vi "New from bytes.vi"(8 "error in":errorcluster, 11 "bytes":u8[](array[numeric]) format="%x") -> (0 "error out":errorcluster, 2 "output cluster":refnum<class "MsgPackString.lvclass">, 3 "remaining bytes":u8[](array[numeric]) format="%x")   [LabVIEW 2020, in "MessagePack.lvlib" / "MsgPackString.lvclass"]
uses:
  MsgPackString/MsgPackString.lvclass
  MsgPackString/MsgPackString.lvclass/MsgPackString.ctl
  <vilib>/Utility/error.llb/Error Cluster From Error Code.vi
  <vilib>/ErrorRing/Error Ring.xnode
  MessagePack.lvlib
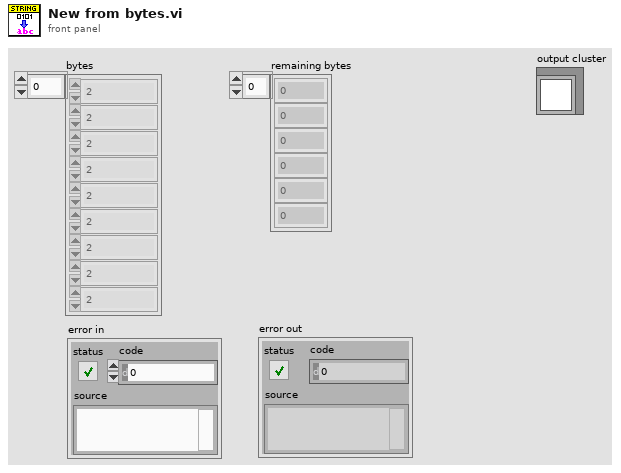
[diagram p1: front panel]
types:
  T1 = typedef "MessagePack.lvlib/MsgPack Object Types.ctl" = enum16{"UNSUPPORTED", "POSINT", "NEGINT", "FIXMAP", "FIXARRAY", "FIXSTR", "NIL", "FALSE", "TRUE", "BIN8", "BIN16", "BIN32", "EXT8", "EXT16", "EXT32", "FLOAT32", "FLOAT64", "UINT8", "UINT16", "UINT32", "UINT64", "INT8", "INT16", "INT32", "INT64", "FIXEXT1", "FIXEXT2", "FIXEXT4", "FIXEXT8", "FIXEXT16", "STR8", "STR16", "STR32", "ARRAY16", "ARRAY32", "MAP16", "MAP32"}
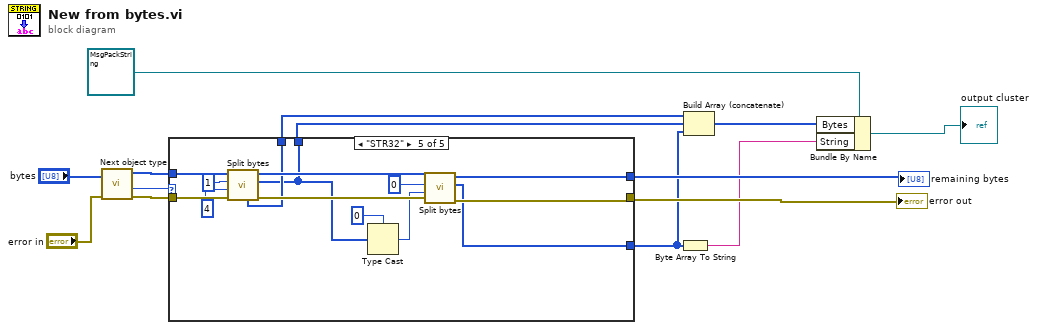
[diagram p0: block diagram]
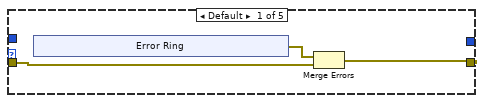
[diagram p2: hidden frame]
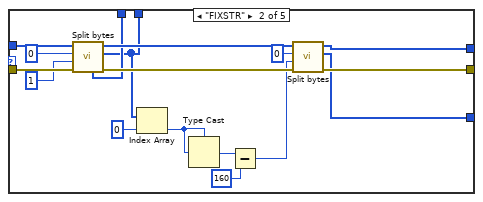
[diagram p3: hidden frame]
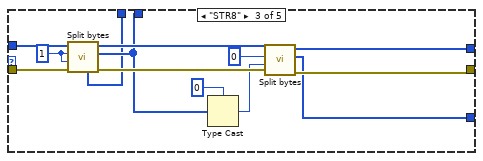
[diagram p4: hidden frame]
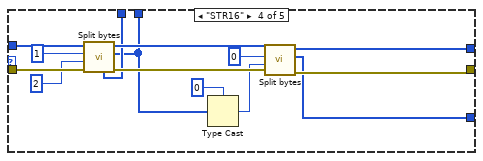
[diagram p5: hidden frame]
diagram:
  n1 = call "Next object type.vi"("error in (no error)"="error in", "Bytes in"="bytes") -> ("error out"=w12:errorcluster, "MsgPack Type"=w7:T1, "Bytes out"=w11:u8[])  [unwired: 6 in, 1 out]
  n2 = case shown="\"STR32\"" w7 {
    tunnel: w12 -> [w17 w38 w50 w64 w78]
    tunnel: [w15 w28 w43 w56 w70] -> w9
    tunnel: w11 -> [_ w37 w51 w65 w79]
    tunnel: [_ w29 w44 w57 w71] -> w10
    tunnel: [_ w26 w42 w54 w68] -> w2
    tunnel: [_ w23 w39 w53 w67] -> w3
    tunnel: [_ w22 w40 w52 w66] -> w1
    frame Default {
      n3 = xnode "Error Ring"() -> ("error out"=w16:errorcluster)
      n4 = Merge Errors(w16, w17) -> (w15:errorcluster)
    }
    frame "FIXSTR" {
      n5 = call "Split bytes.vi"("error in"=w38, "Count"=1, "Start index"=0, "bytes in"=w37) -> ("error out"=w27:errorcluster, "selected bytes"=w22:u8[], "remaining bytes"=w30:u8[], "before bytes"=w23:u8[])  [unwired: 4 in]
      n6 = Index Array(array=w22, index=0) -> (element=w34:u8)
      n7 = Type Cast(type=w34, x=w34) -> (*(type *) &x=w33:u8)
      n8 = Subtract(x=w33, y=u8 160) -> (x-y=w25:u8)
      n9 = call "Split bytes.vi"("error in"=w27, "Count"=w25, "Start index"=0, "bytes in"=w30) -> ("error out"=w28:errorcluster, "selected bytes"=w26:u8[], "remaining bytes"=w29:u8[])  [unwired: 4 in, 1 out]
    }
    frame "STR8" {
      w41 = 1 ("Start index")
      n10 = call "Split bytes.vi"("error in"=w50, "Count"=w41, "Start index"=w41, "bytes in"=w51) -> ("error out"=w47:errorcluster, "selected bytes"=w40:u8[], "remaining bytes"=w48:u8[], "before bytes"=w39:u8[])  [unwired: 4 in]
      n11 = Type Cast(type=u8 0, x=w40) -> (*(type *) &x=w45:u8)
      n12 = call "Split bytes.vi"("error in"=w47, "Count"=w45, "Start index"=0, "bytes in"=w48) -> ("error out"=w43:errorcluster, "selected bytes"=w42:u8[], "remaining bytes"=w44:u8[])  [unwired: 4 in, 1 out]
    }
    frame "STR16" {
      n13 = call "Split bytes.vi"("error in"=w64, "Count"=2 ("End index"), "Start index"=1, "bytes in"=w65) -> ("error out"=w60:errorcluster, "selected bytes"=w52:u8[], "remaining bytes"=w61:u8[], "before bytes"=w53:u8[])  [unwired: 4 in]
      n14 = Type Cast(type=u16 0, x=w52) -> (*(type *) &x=w58:u16)
      n15 = call "Split bytes.vi"("error in"=w60, "Count"=w58, "Start index"=0, "bytes in"=w61) -> ("error out"=w56:errorcluster, "selected bytes"=w54:u8[], "remaining bytes"=w57:u8[])  [unwired: 4 in, 1 out]
    }
    frame "STR32" {
      n16 = call "Split bytes.vi"("error in"=w78, "Count"=4 ("End index"), "Start index"=1, "bytes in"=w79) -> ("error out"=w74:errorcluster, "selected bytes"=w66:u8[], "remaining bytes"=w75:u8[], "before bytes"=w67:u8[])  [unwired: 4 in]
      n17 = Type Cast(type=u32 0, x=w66) -> (*(type *) &x=w72:u32)
      n18 = call "Split bytes.vi"("error in"=w74, "Count"=w72, "Start index"=0, "bytes in"=w75) -> ("error out"=w70:errorcluster, "selected bytes"=w68:u8[], "remaining bytes"=w71:u8[])  [unwired: 4 in, 1 out]
    }
  }
  "error out" <- w9
  "remaining bytes" <- w10
  n19 = Byte Array To String(unsigned byte array=w2) -> (string=w6:string)
  n20 = Build Array (concatenate)(w3, w1, w2) -> (w4:u8[])
  n21 = Bundle By Name(cluster=refnum<class "MsgPackString.lvclass"> refnum ("MessagePack.lvlib:MsgPackString.lvclass"), "Bytes"=w4, "String"=w6) -> (→"output cluster":refnum<class "MsgPackString.lvclass">)
